vi "test sym danych Q.vi"() -> ()   [LabVIEW 2015, in "Biblioteka moduł map v3.lvlib" / "Generatory_symulatory.lvlib"]
uses:
  Testowe/Generatory_symulatory.lvlib
  Zmienne/Lokalizacja GPS/longitude Quadron.vi
  Zmienne/Lokalizacja GPS/latitude Quadron.vi
  Zmienne/Lokalizacja GPS/latitude.vi
  Zmienne/Lokalizacja GPS/longitude.vi
  Zmienne/Lokalizacja GPS/Longitude dron 1.vi
  Zmienne/Lokalizacja GPS/Latitude dron 1.vi
  Zmienne/Lokalizacja GPS/Latitude dron 2.vi
  Zmienne/Lokalizacja GPS/Longitude dron 2.vi
  Zmienne/Lokalizacja GPS/Latitude Sparus.vi
  Zmienne/Lokalizacja GPS/Longitude Sparus.vi
  Zmienne/Lokalizacja GPS/Lokalizacja GPS.lvlib
panel:
  in  "Longitude Sparus":dbl format="%.5g"
  in  "Latitude Sparus":dbl format="%.5g"
  in  "Longitude dron 2":dbl format="%.5g"
  in  "Latitude dron 2":dbl format="%.5g"
  in  "Latitude dron 1":dbl format="%.5g"
  in  "Longitude dron 1":dbl format="%.5g"
  in  "stop":bool
  in  "Longitude":dbl format="%.5g"
  in  "latitude":dbl format="%.5g"
  in  "latitude Quadron":dbl format="%.5g"
  in  "Longitude Quadron":dbl format="%.5g"
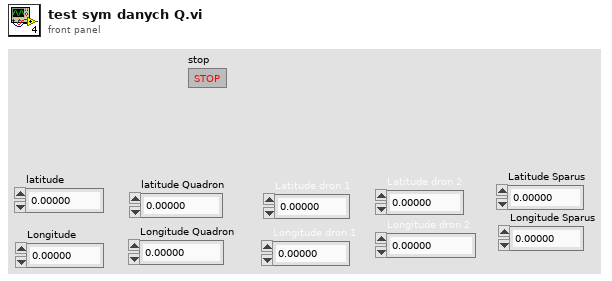
[diagram p1: front panel]
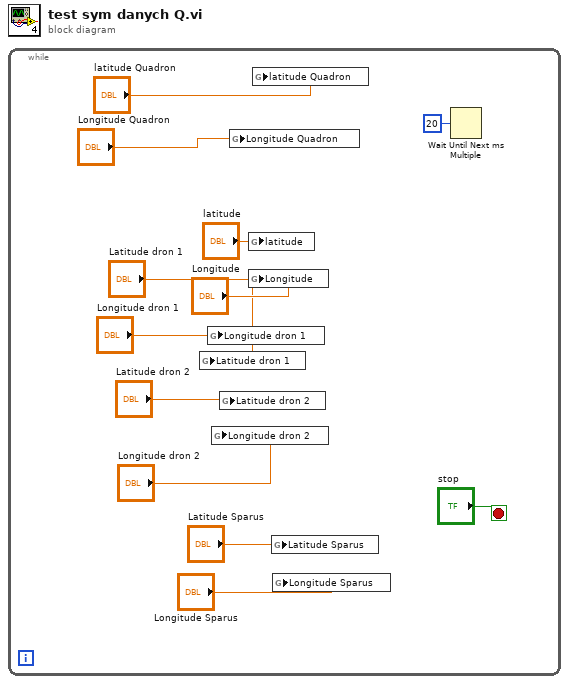
[diagram p0: block diagram]
diagram:
  n1 = while {
    stop <- "stop" stop-if-true
    n2 = global write "Latitude dron 1.vi" "Latitude dron 1"("Latitude dron 1") -> ()
    n3 = global write "Longitude dron 1.vi" "Longitude dron 1"("Longitude dron 1") -> ()
    n4 = global write "Longitude dron 2.vi" "Longitude dron 2"("Longitude dron 2") -> ()
    n5 = global write "Latitude dron 2.vi" "Latitude dron 2"("Latitude dron 2") -> ()
    n6 = global write "longitude Quadron.vi" "Longitude Quadron"("Longitude Quadron") -> ()
    n7 = global write "latitude.vi" "latitude"("latitude") -> ()
    n8 = global write "longitude.vi" "Longitude"("Longitude") -> ()
    n9 = global write "latitude Quadron.vi" "latitude Quadron"("latitude Quadron") -> ()
    n10 = global write "Latitude Sparus.vi" "Latitude Sparus"("Latitude Sparus") -> ()
    n11 = global write "Longitude Sparus.vi" "Longitude Sparus"("Longitude Sparus") -> ()
    n12 = Wait Until Next ms Multiple(millisecond multiple=u32 20) -> ()  [unwired: 1 out]
  }
